vi "Goto.vi"(3 "TranslationStages.lvclass":refnum<class "TranslationStages.lvclass">, 7 "Speed":i32, 8 "error in (no error)":errorcluster, 9 "Direction":enum16{""}(ring), 10 "New Position":enum16{""}(ring)) -> (0 "error out":errorcluster, 11 "TranslationStages.lvclass":refnum<class "TranslationStages.lvclass">)   [LabVIEW 2023, in "TranslationStages.lvclass"]
uses:
  TranslationStages.lvclass
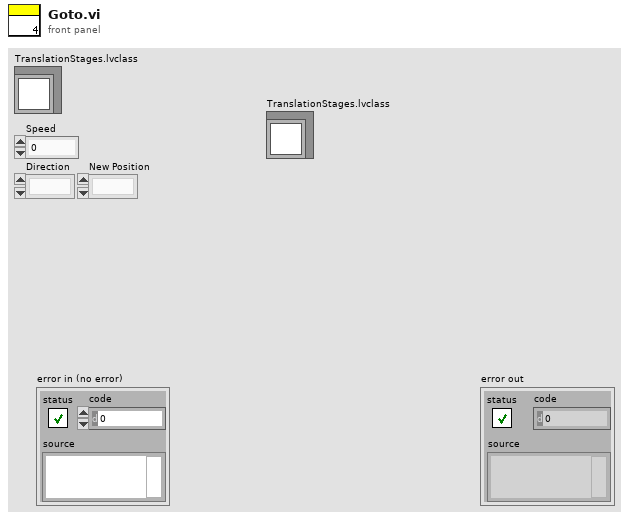
[diagram p1: front panel]
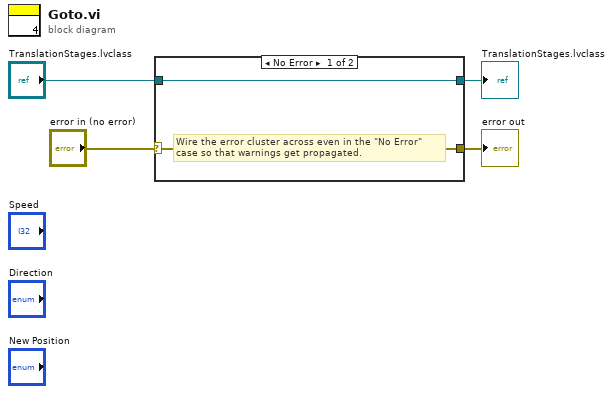
[diagram p0: block diagram]
diagram:
  n1 = case shown="No Error" "error in (no error)" {
    selector: "error in (no error)" -> [w5 w8]
    tunnel: [w5 w8] -> w3
    tunnel: [w6 w7] -> w1
    tunnel: "TranslationStages.lvclass" -> [w6 w7]
    frame No Error {
      # "Wire the error cluster across even in the \"No Error\"\ncase so that warnings get propagated."
    }
    frame Error {
    }
  }
  "error out" <- w3
  "TranslationStages.lvclass" <- w1
